vi "Build Description String.vi"(8 "error in (no error)":errorcluster, 11 "Window Action in":refnum<class "Window Action.lvclass">) -> (0 "error out":errorcluster, 1 "Description":string, 2 "Subtype String":string, 3 "Window Action out":refnum<class "Window Action.lvclass">)   [LabVIEW 2020, in "MacroAssert.lvlib" / "Window Action.lvclass"]
doc: "Builds a string to describe what <B>Step</B> does."
uses:
  Window Action.lvclass
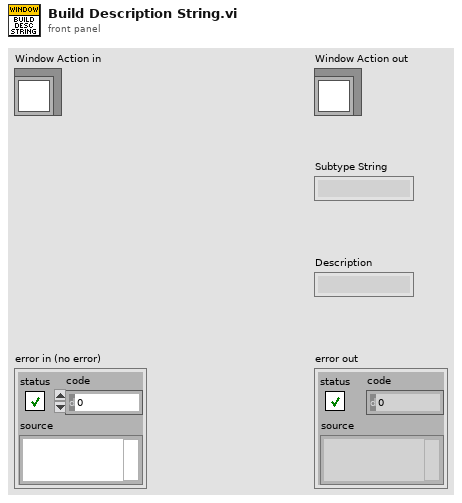
[diagram p1: front panel]
types:
  T1 = typedef "MacroAssert.lvlib/Window Action.lvclass/Window Action Type.ctl" = enum16{"Maximize Window", "Restore Window", "Minimize Window", "Close Window", "Bring Window to Front", "Send Window to Back"}
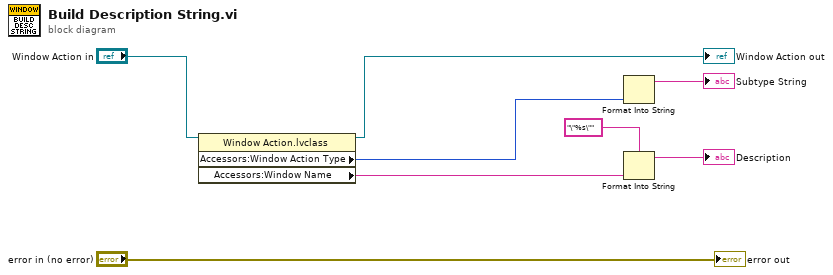
[diagram p0: block diagram]
diagram:
  n1 = property class="Window Action.lvclass"(reference="Window Action in") -> (reference out=→"Window Action out":refnum<class "Window Action.lvclass">, "Accessors:Window Action Type"=w1:T1, "Accessors:Window Name"=w3:string)  [unwired: 1 in, 1 out]
  n2 = Format Into String(w1) -> (resulting string=→"Subtype String":string)  [unwired: 3 in, 1 out]
  n3 = Format Into String(format string="\"%s\"", w3) -> (resulting string=→"Description":string)  [unwired: 2 in, 1 out]
  "error out" <- "error in (no error)"
